vi "Modified Sync Filter w_a(x).vi"(0 "x(i)":dbl, 2 "alpha":dbl) -> (7 "w_a(x)":dbl)   [LabVIEW 2021, in "Math.lvlib"]
uses:
  Math.lvlib
panel:
  # "see the License on the block diagram (Ctrl+E or Window:Show Block Diagram)"
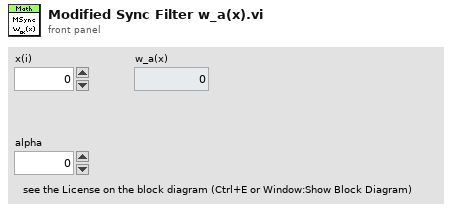
[diagram p1: front panel]
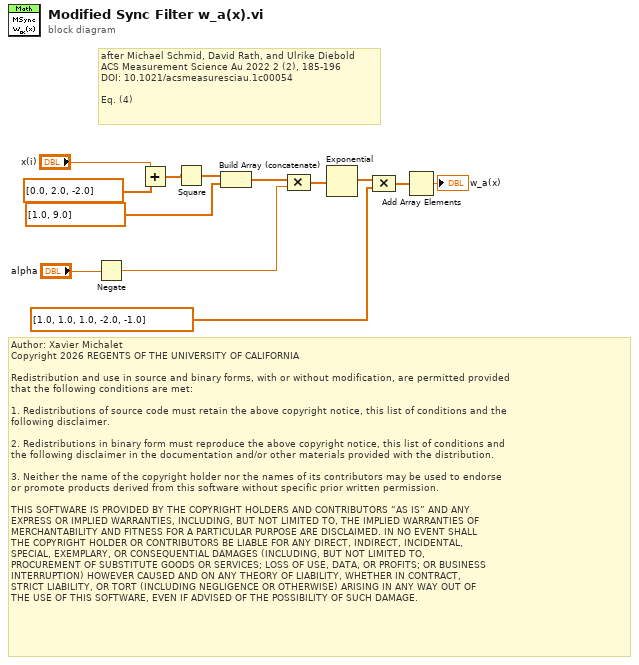
[diagram p0: block diagram]
diagram:
  # "Author: Xavier Michalet\nCopyright 2026 REGENTS OF THE UNIVERSITY OF CALIFORNIA\n\nRedistribution and use in source and binary forms, with or without modification, are permitted provided\nthat the following conditions are met:\n\n1. Redistributions of source code must retain the above copyright notice, this list of conditions and the\nfollowing disclaimer.\n\n2. Redistributions in binary form must reproduce the above copyright notice, this list of conditions and\nthe following disclaimer in the documentation and/or other materials provided with the distribution.\n\n3. Neither the name of the copyright holder nor the names of its contributors may be used to endorse \nor promote products derived from this software without specific prior written permission.\n\nTHIS SOFTWARE IS PROVIDED BY THE COPYRIGHT HOLDERS AND CONTRIBUTORS “AS IS” AND ANY \nEXPRESS OR IMPLIED WARRANTIES, INCLUDING, BUT NOT LIMITED TO, THE IMPLIED WARRANTIES OF\nMERCHANTABILITY AND FITNESS FOR A PARTICULAR PURPOSE ARE DISCLAIMED. IN NO EVENT SHALL\nTHE COPYRIGHT HOLDER OR CONTRIBUTORS BE LIABLE FOR ANY DIRECT, INDIRECT, INCIDENTAL, \nSPECIAL, EXEMPLARY, OR CONSEQUENTIAL DAMAGES (INCLUDING, BUT NOT LIMITED TO, \nPROCUREMENT OF SUBSTITUTE GOODS OR SERVICES; LOSS OF USE, DATA, OR PROFITS; OR BUSINESS\nINTERRUPTION) HOWEVER CAUSED AND ON ANY THEORY OF LIABILITY, WHETHER IN CONTRACT, \nSTRICT LIABILITY, OR TORT (INCLUDING NEGLIGENCE OR OTHERWISE) ARISING IN ANY WAY OUT OF\nTHE USE OF THIS SOFTWARE, EVEN IF ADVISED OF THE POSSIBILITY OF SUCH DAMAGE."
  # "after Michael Schmid, David Rath, and Ulrike Diebold\nACS Measurement Science Au 2022 2 (2), 185-196\nDOI: 10.1021/acsmeasuresciau.1c00054\n\nEq. (4)"
  n1 = Negate(x="alpha") -> (-x=w5:dbl)
  n2 = Add(x="x(i)", y=dbl[] [0.0, 2.0, -2.0]) -> (x+y=w11:dbl[])
  n3 = Square(x=w11) -> (x^2=w10:dbl[])
  n4 = Build Array (concatenate)(w10, dbl[] [1.0, 9.0]) -> (w7:dbl[])
  n5 = Compound Arithmetic op=MULTIPLY(w7, w5) -> (w8:dbl[])
  n6 = Exponential(1:w8) -> (0:w4:dbl[])
  n7 = Compound Arithmetic op=MULTIPLY(w4, dbl[] [1.0, 1.0, 1.0, -2.0, -1.0]) -> (w2:dbl[])
  n8 = Add Array Elements(numeric array=w2) -> (sum=→"w_a(x)":dbl)
